vi "Asynchronous Call and Collect (Using Option 0x40).vi"() -> ()   [LabVIEW 2016]
doc: "This example uses the Open VI Reference option 0x40 in conjunction with asynchronous VI calls.\n\nThe Open VI Reference option 0x40 will enable simultaneous calls on reentrant VIs. This allows one VI Reference to be used to call multiple reentrant instances of the target VI simultaneously where the execution of the target VI instances will happen in parallel.\n\nThis example demonstrates that use of option 0x40 to reduce the total execution time of the multiple calls. When option 0x40 is passed into Open VI Reference, the asynchronous calls can occur in parallel. However, if 0x40 is not passed in, the execution of the calls will be serialized.\n\nIn this example, the target VI will run for 100 ms a piece. If option 0x40 is passed into the Open VI Reference, the calls can take place simultaneously. If option 0x40 is not passed in, the calls will serialize."
panel:
  out "Elapsed time with option 0x40":u32
  out "Elapsed time without option 0x40":u32
  # "Overview: Demonstrates the use of option 0x40 with Asynchronous VI Calls.\nInstructions:\nRun the VI. Observe the benchmark values below. See the block diagram for more information."
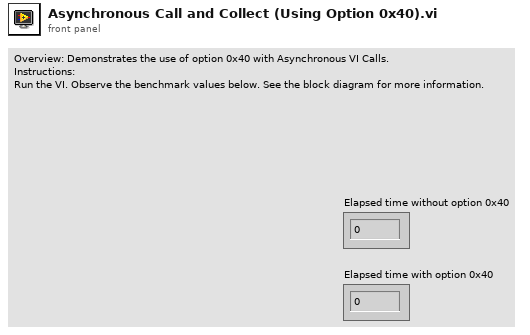
[diagram p1: front panel]
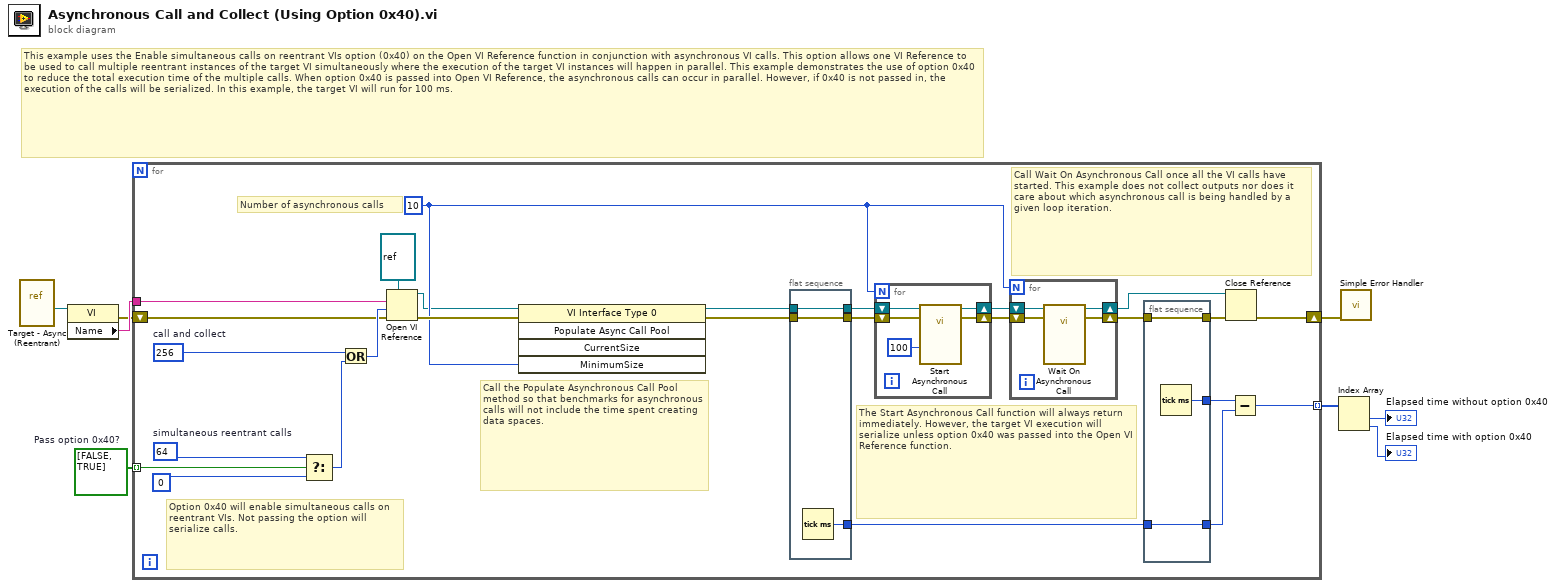
[diagram p0: block diagram]
diagram:
  w8 = bool[] [FALSE, TRUE]  # Pass option 0x40?
  # "This example uses the Enable simultaneous calls on reentrant VIs option (0x40) on the Open VI Reference function in conjunction with asynchronous VI calls. This option allows one VI Reference to be used to call multiple reentrant instances of the target VI simultaneously where the execution of the target VI instances will happen in parallel. This example demonstrates the use of option 0x40 to reduce the total execution time of the multiple calls. When option 0x40 is passed into Open VI Reference, the asynchronous calls can occur in parallel. However, if 0x40 is not passed in, the execution of the calls will be serialized. In this example, the target VI will run for 100 ms."
  n1 = vi-ref "Target - Async (Reentrant).vi"() -> (w5:refnum<vi>)
  n2 = property class="VI"(reference=w5) -> (error out=w2:errorcluster, "Name"=w4:string)  [unwired: 1 in, 1 out]
  n3 = for {
    tunnel: w8 -> [w18] mode=indexing
    tunnel: [w17] -> w7 mode=indexing
    tunnel: w4 -> [w16]
    shift-right: [w33] -> w1
    shift-left: w2 -> [w11]
    w26 = 64  # simultaneous reentrant calls
    w12 = 10
    w29 = 256  # call and collect
    # "Call the Populate Asynchronous Call Pool method so that benchmarks for asynchronous calls will not include the time spent creating data spaces."
    # "The Start Asynchronous Call function will always return immediately. However, the target VI execution will serialize unless option 0x40 was passed into the Open VI Reference function."
    # "Number of asynchronous calls"
    # "Call Wait On Asynchronous Call once all the VI calls have started. This example does not collect outputs nor does it care about which asynchronous call is being handled by a given loop iteration."
    # "Option 0x40 will enable simultaneous calls on reentrant VIs. Not passing the option will serialize calls."
    n4 = Select(t=w26, s=w18, f=0 ("options")) -> (s? t:f=w25:i32)
    n5 = Or(x=w29, y=w25) -> (x .or. y?=w28:i32)
    n6 = Open VI Reference(type specifier VI Refnum (for type only)=refnum<vi> refnum, vi path=w16, options=w28, error in (no error)=w11) -> (vi reference=w10:refnum<vi>, error out=w15:errorcluster)  [unwired: 2 in]
    n7 = invoke class="VI Interface Type 0" method="Populate Async Call Pool"(reference=w10, error in=w15, "MinimumSize"=w12) -> (reference out=w13:refnum<vi>, error out=w14:errorcluster)  [unwired: 2 in, 3 out]
    n8 = flat-sequence {
      tunnel: [w40] -> w24
      tunnel: w14 -> [w40]
      tunnel: [w39] -> w19
      tunnel: [w38] -> w9
      tunnel: w13 -> [w38]
      frame #0 {
        n9 = Tick Count (ms)() -> (millisecond timer value=w39:u32)
      }
    }
    n10 = for {
      N: w12 -> [_]
      shift-right: [w46] -> w31
      shift-left: w24 -> [w48]
      shift-right: [w47] -> w32
      shift-left: w9 -> [w49]
      n11 = call-by-ref "Start Asynchronous Call"(reference=w49, error in=w48, "Wait (Milliseconds)"=u32 100) -> (reference out=w47:refnum<vi>, error out=w46:errorcluster)  [unwired: 10 in, 1 out]
    }
    n12 = for {
      N: w12 -> [_]
      shift-right: [w41] -> w23
      shift-left: w31 -> [w43]
      shift-right: [w42] -> w30
      shift-left: w32 -> [w44]
      n13 = call-by-ref "Wait On Asynchronous Call"(reference=w44, error in=w43) -> (reference out=w42:refnum<vi>, error out=w41:errorcluster)  [unwired: 11 in, 1 out]
    }
    n14 = flat-sequence {
      tunnel: [w37] -> w22
      tunnel: w23 -> [w37]
      tunnel: [w36] -> w21
      tunnel: [w35] -> w20
      tunnel: w19 -> [w35]
      frame #0 {
        n15 = Tick Count (ms)() -> (millisecond timer value=w36:u32)
      }
    }
    n16 = Close Reference(reference=w30, error in (no error)=w22) -> (error out=w33:errorcluster)
    n17 = Subtract(x=w21, y=w20) -> (x-y=w17:u32)
  }
  n18 = Index Array(array=w7) -> (element #1=→"Elapsed time without option 0x40":u32, element #2=→"Elapsed time with option 0x40":u32)  [unwired: 2 in]
  n19 = call <vilib>:"Simple Error Handler.vi"("error in (no error)"=w1) -> ()  [unwired: 4 in, 5 out]
